vi "blink red.vi"(2 "error in":errorcluster, 3 "task in\n(diody dolne)":refnum<k21>) -> (0 "error out":errorcluster, 1 "task out\n(diody dolne)":refnum<k21>)   [LabVIEW 2023]
uses:
  <vilib>/DAQmx/write.llb/DAQmx Write (Digital 1D Bool 1Chan 1Samp).vi
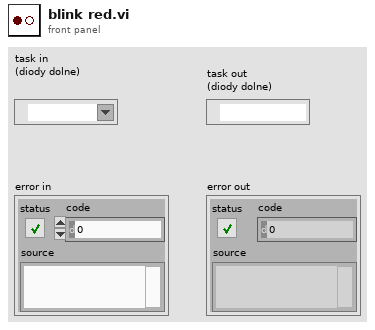
[diagram p1: front panel]
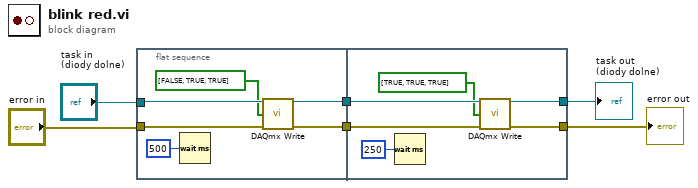
[diagram p0: block diagram]
diagram:
  n1 = flat-sequence {
    tunnel: "task in\n(diody dolne)" -> [w12]
    tunnel: [w11] -> w6
    tunnel: "error in" -> [w10]
    tunnel: [w9] -> w5
    tunnel: w6 -> [w18]
    tunnel: [w17] -> w2
    tunnel: w5 -> [w16]
    tunnel: [w15] -> w4
    frame #0 {
      n2 = Wait (ms)(milliseconds to wait=u32 500) -> ()  [unwired: 1 out]
      n3 = call-poly <vilib>:"DAQmx Write.vi"("task/channels in"=w12, "data"=bool[] [FALSE, TRUE, TRUE], "error in"=w10) -> ("task out"=w11:refnum<k21>, "error out"=w9:errorcluster)  [unwired: 10 in, 1 out]
    }
    frame #1 {
      n4 = Wait (ms)(milliseconds to wait=u32 250) -> ()  [unwired: 1 out]
      n5 = call-poly <vilib>:"DAQmx Write.vi"("task/channels in"=w18, "data"=bool[] [TRUE, TRUE, TRUE], "error in"=w16) -> ("task out"=w17:refnum<k21>, "error out"=w15:errorcluster)  [unwired: 10 in, 1 out]
    }
  }
  "error out" <- w4
  "task out\n(diody dolne)" <- w2
